vi "SP Calculate SXY.vi"(10 "TP Array (TXX, TXY, TYX, TYY)":cdb[](array[numeric])) -> (2 "SXY":cdb)   [LabVIEW 2011]
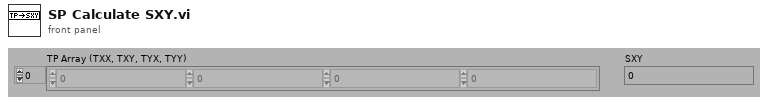
[diagram p1: front panel]
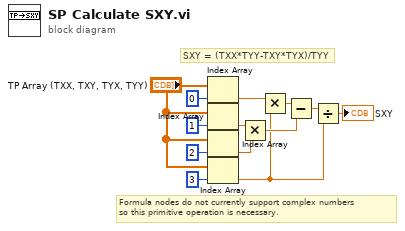
[diagram p0: block diagram]
diagram:
  # "SXY = (TXX*TYY-TXY*TYX)/TYY"
  # "Formula nodes do not currently support complex numbers\nso this primitive operation is necessary."
  n1 = Index Array(array="TP Array (TXX, TXY, TYX, TYY)", index=0) -> (element=w8:cdb)
  n2 = Index Array(array="TP Array (TXX, TXY, TYX, TYY)", index=1) -> (element=w7:cdb)
  n3 = Index Array(array="TP Array (TXX, TXY, TYX, TYY)", index=2) -> (element=w4:cdb)
  n4 = Index Array(array="TP Array (TXX, TXY, TYX, TYY)", index=3) -> (element=w1:cdb)
  n5 = Multiply(x=w7, y=w4) -> (x*y=w5:cdb)
  n6 = Multiply(x=w8, y=w1) -> (x*y=w6:cdb)
  n7 = Subtract(x=w6, y=w5) -> (x-y=w3:cdb)
  n8 = Divide(x=w3, y=w1) -> (x/y=→"SXY":cdb)
